vi "_rsscope Coercing Warning.vi"(7 "In Range?":bool, 8 "error in (no error)":errorcluster, 11 "VISA resource name":refnum<visa-resource-name>) -> (0 "error out":errorcluster, 3 "VISA resource name out":refnum<visa-resource-name>)   [LabVIEW 2014]
doc: "This VI updates error cluster with a warning code if any of the user input values have been coerced."
uses:
  rsidr_core.llb/type_Error_Codes.ctl
  rsidr_core.llb/rsscope_rsidr_core.lvlib
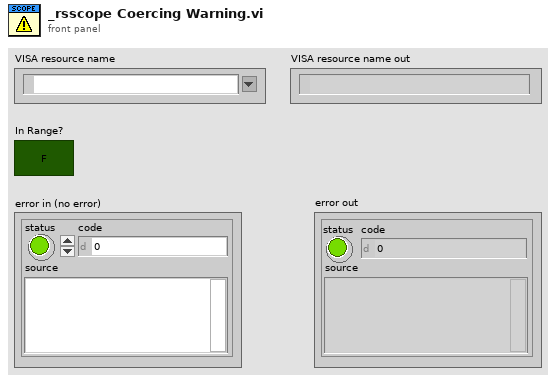
[diagram p1: front panel]
types:
  T1 = typedef "rsscope_rsidr_core.lvlib/type_Error_Codes.ctl" = enum16{"No_error", "VISA_err_ResourceNotFound", "VISA_err_Timeout", "VISA_warn_MoreDataAvailable", "RS_err_MissingCallback", "RS_err_InvalidAttribute", "RS_err_InvalidValue", "RS_err_UnknownResource", "RS_err_AlreadyInitialized", "RS_err_InstrumentStatus", "RS_err_BadRepCapName", "RS_err_TypesMismatch", "RS_err_ValueNotSupported", "RS_err_InvalidRngTable", "RS_err_IDqueryFail", "RS_err_UnexpResponse", "VISA_warn_ConfigNotLoaded", "RS_err_AttributeNotReadable", "RS_err_AttributeNotWritable", "RS_err_InstrumentType", "RS_err_InstrumentOption", "VISA_err_InvalidSize", "RS_err_ReliabilityIndicator", "VISA_warn_UnknownStatus", "VISA_warn_TermCharRead", "VISA_err_IO_error", "RS_err_FunctionNotSupported", "VISA_warn_QueueEmpty"}
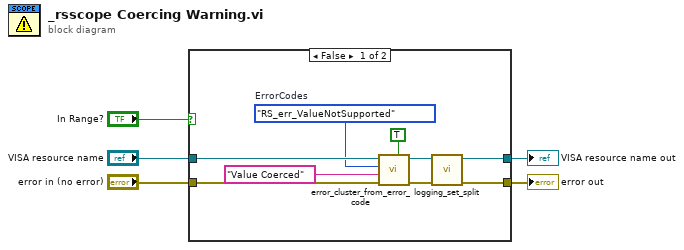
[diagram p0: block diagram]
diagram:
  n1 = case shown="False" "In Range?" {
    tunnel: "error in (no error)" -> [w12 w16]
    tunnel: "VISA resource name" -> [w11 w15]
    tunnel: [w7 w16] -> w3
    tunnel: [w6 w15] -> w2
    frame False {
      w10 = type_Error_Codes."RS_err_ValueNotSupported"  # ErrorCodes
      n2 = call "error_cluster_from_error_code.vi"("Is Warning (False)"=TRUE ("is warning? (False)"), "error in"=w12, "Error Message (\"\")"="Value Coerced" ("error message (\"\")"), "Error Enum in"=w10, "VISA resource name"=w11) -> ("error out"=w9:errorcluster, "VISA resource name out"=w8:refnum<visa-resource-name>)  [unwired: 5 in]
      n3 = call "logging_set_split.vi"("error in"=w9, "VISA resource name"=w8) -> ("error out"=w7:errorcluster, "VISA resource name out"=w6:refnum<visa-resource-name>)  [unwired: 8 in]
    }
    frame True {
    }
  }
  "error out" <- w3
  "VISA resource name out" <- w2
